vi "Start Totalize Cycle.vi"(7 "Period Seconds (0)":i32, 8 "error in (no error)":errorcluster, 9 "Period Minutes (1)":i32=1, 10 "Period Hours (0)":i32, 11 "VISA resource name":refnum<visa-resource-name>) -> (0 "error out":errorcluster, 3 "VISA resource name out":refnum<visa-resource-name>)   [LabVIEW 2023, in "Fluke Molbox 1 Plus.lvlib"]
doc: "Start a new totalize cycle. The totalizing cycle accumulates the total mass or volume flowed over a set period, or the user can stop the cycle early if desired to use a shorter period than specified."
uses:
  Fluke Molbox 1 Plus.lvlib
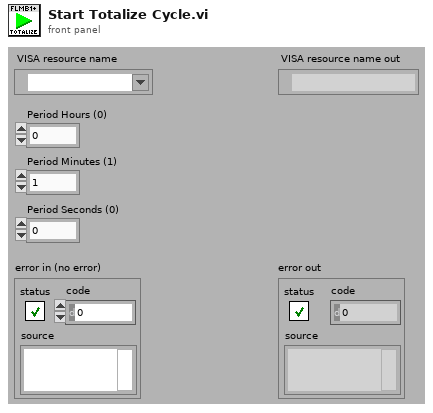
[diagram p1: front panel]
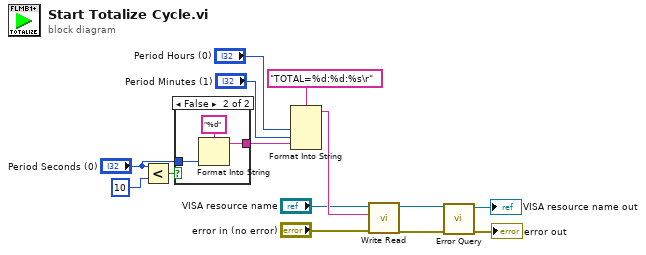
[diagram p0: block diagram]
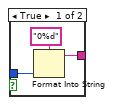
[diagram p2: hidden frame]
diagram:
  n1 = Less?(x="Period Seconds (0)", y=u32 10) -> (x < y?=w13:bool)
  n2 = case shown="False" w13 {
    tunnel: "Period Seconds (0)" -> [w17 w20]
    tunnel: [w15 w18] -> w9
    frame True {
      n3 = Format Into String(format string="0%d", w17) -> (resulting string=w15:string)  [unwired: 2 in, 1 out]
    }
    frame False {
      n4 = Format Into String(format string="%d", w20) -> (resulting string=w18:string)  [unwired: 2 in, 1 out]
    }
  }
  n5 = Format Into String(format string="TOTAL=%d:%d:%s\r", "Period Hours (0)", "Period Minutes (1)", w9) -> (resulting string=w2:string)  [unwired: 2 in, 1 out]
  n6 = call "Write Read.vi"("error in (no error)"="error in (no error)", "Write String"=w2, "VISA resource name"="VISA resource name") -> ("error out"=w4:errorcluster, "VISA resource name out"=w5:refnum<visa-resource-name>)  [unwired: 6 in, 1 out]
  n7 = call "Error Query.vi"("error in (no error)"=w4, "VISA resource name"=w5) -> ("error out"=→"error out":errorcluster, "VISA resource name out"=→"VISA resource name out":refnum<visa-resource-name>)  [unwired: 6 in, 2 out]
